vi "Part 1.vi"(11 "Input":string) -> (3 "Output":i64)   [LabVIEW 2021]
uses:
  <userlib>/_OpenG.lib/string/string.llb/Convert EOLs (String)__ogtk.vi
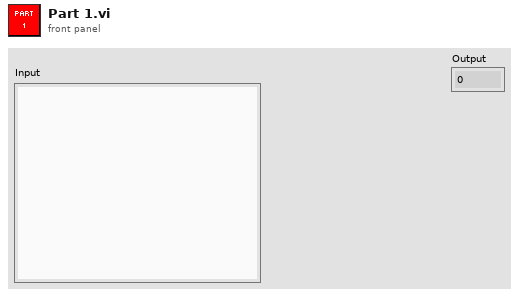
[diagram p1: front panel]
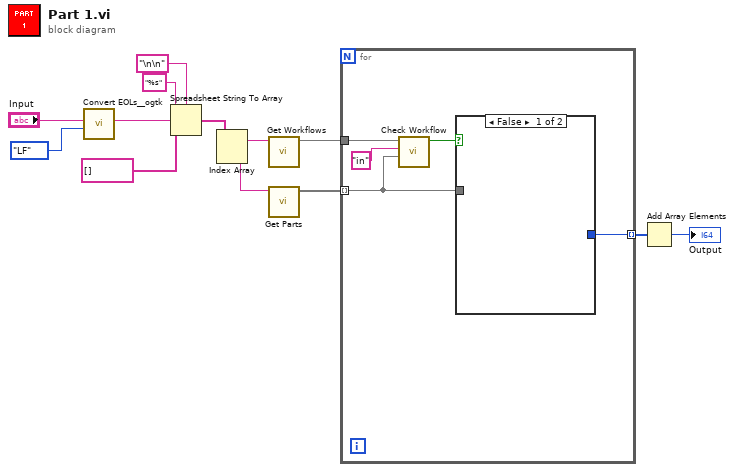
[diagram p0: block diagram]
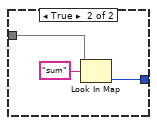
[diagram p2: hidden frame]
diagram:
  n1 = call-poly <userlib>:"Convert EOLs__ogtk.vi"("Convert to:"=enum16{"CR", "LF", "CRLF"}."LF", "String in"="Input") -> ("String out"=w9:string)  [unwired: 9 in]
  n2 = Spreadsheet String To Array(delimiter (Tab)="\n\n", format string="%s", spreadsheet string=w9, array type (2D Dbl)=string[] []) -> (array=w7:string[])
  n3 = Index Array(array=w7) -> (element #1=w2:string, element #2=w6:string)  [unwired: 2 in]
  n4 = call "Get Workflows.vi"("Workflows In"=w2) -> ("Workflow Map"=w1:map{string, string[]})  [unwired: 10 in]
  n5 = call "Get Parts.vi"("Part list"=w6) -> ("Parts"=w4:map{string, i64}[])  [unwired: 10 in]
  n6 = for {
    tunnel: w4 -> [w15] mode=indexing
    tunnel: [w18] -> w3 mode=indexing
    tunnel: w1 -> [w17]
    n7 = call "Check Workflow.vi"("Part In"=w15, "Current  Workflow"="in", "Workflow Map"=w17) -> ("Accepted?"=w16:bool)  [unwired: 8 in]
    n8 = case shown="False" w16 {
      tunnel: w15 -> [_ w21]
      tunnel: [_ w19] -> w18
      frame False {
      }
      frame True {
        n9 = Look In Map(map=w21, key="sum") -> (value=w19:i64)  [unwired: 1 in, 1 out]
      }
    }
  }
  n10 = Add Array Elements(numeric array=w3) -> (sum=→"Output":i64)
